vi "SendUpstreamMessage.vi"(8 "error in (no error)":errorcluster, 10 "UpstreamMsg":refnum<class "UpstreamMsgParent.lvclass">, 11 "ServiceManager-DebugView in":refnum<class "ServiceManager-DebugView.lvclass">) -> (0 "error out":errorcluster, 3 "ServiceManager-DebugView out":refnum<class "ServiceManager-DebugView.lvclass">)   [LabVIEW 2020, in "ServiceManager-DebugView.lvlib" / "ServiceManager-DebugView.lvclass"]
uses:
  ServiceManager-DebugView.lvclass
  UpstreamMsg/UpstreamMsgParent/UpstreamMsgParent.lvclass
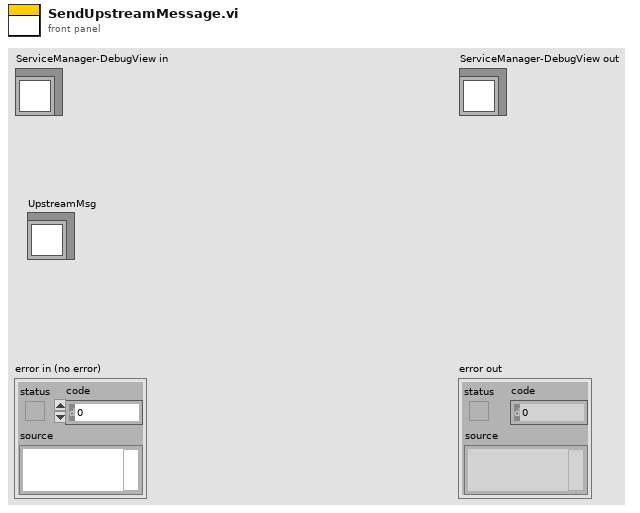
[diagram p1: front panel]
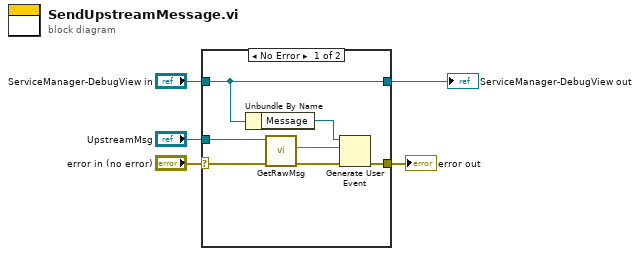
[diagram p0: block diagram]
diagram:
  n1 = case shown="No Error" "error in (no error)" {
    selector: "error in (no error)" -> [w11 w13]
    tunnel: "UpstreamMsg" -> [w12 _]
    tunnel: "ServiceManager-DebugView in" -> [w10 w14]
    tunnel: [w10 w14] -> w2
    tunnel: [w6 w13] -> w1
    frame No Error {
      n2 = Unbundle By Name(w10) -> ("Message"=w7:refnum<user-event>)
      n3 = call-dynamic "GetRawMsg.vi"("error in (no error)"=w11, "UpstreamMsgParent in"=w12) -> ("error out"=w9:errorcluster, "Msg"=w8:string)  [unwired: 7 in, 1 out]
      n4 = Generate User Event(user event=w7, event data cluster=w8, error in=w9) -> (error out=w6:errorcluster)  [unwired: 1 in, 1 out]
    }
    frame Error {
    }
  }
  "error out" <- w1
  "ServiceManager-DebugView out" <- w2
